vi "communicateUDP.vi"(0 "Communication in":refnum<class "Communication.lvclass">, 1 "Replace Now":bool, 2 "FIRASim?":bool=TRUE, 5 "Robots":T1[](array[typedef]), 7 "isMyTeamYellow":bool, 9 "Address:":string="127.0.0.1", 11 "error in (no error)":errorcluster, 12 "Port:":u16=20011, 13 "grSim replacement":cluster{"robots":T2[], "ball":T3}) -> (4 "Communication out":refnum<class "Communication.lvclass">, 15 "error out":errorcluster)   [LabVIEW 2023, in "Communication.lvclass"]
doc: "Transmits the robots commands to grSim using UDP communication."
uses:
  Communication.lvclass
  Paths/grSim Packet Command UDP Test Folder/grSim/grSim RobotReplacement.ctl
  Paths/grSim Packet Command UDP Test Folder/grSim/grSim_BallReplacement.ctl
  Paths/Convert AI Robot to Robot Command Folder/grSim/grSim Robot Command.ctl
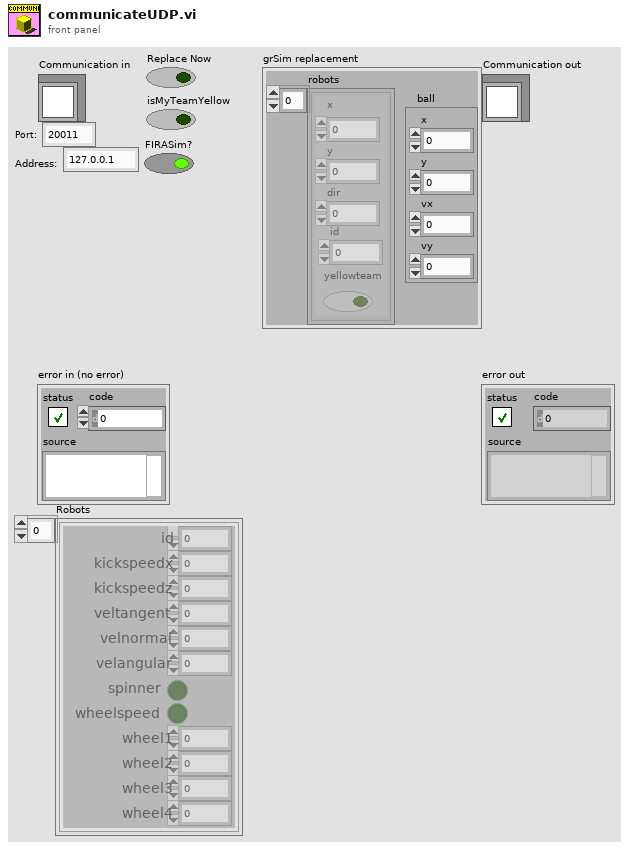
[diagram p1: front panel]
types:
  T1 = typedef "grSim Robot Command.ctl" = cluster{"id":u32, "kickspeedx":sgl, "kickspeedz":sgl, "veltangent":sgl, "velnormal":sgl, "velangular":sgl, "spinner":bool, "wheelspeed":bool, "wheel1":sgl, "wheel2":sgl, "wheel3":sgl, "wheel4":sgl}
  T2 = typedef "grSim RobotReplacement.ctl" = cluster{"x":dbl, "y":dbl, "dir":dbl, "yellowteam":bool, "id":u32}
  T3 = typedef "grSim_BallReplacement.ctl" = cluster{"x":dbl, "y":dbl, "vx":dbl, "vy":dbl}
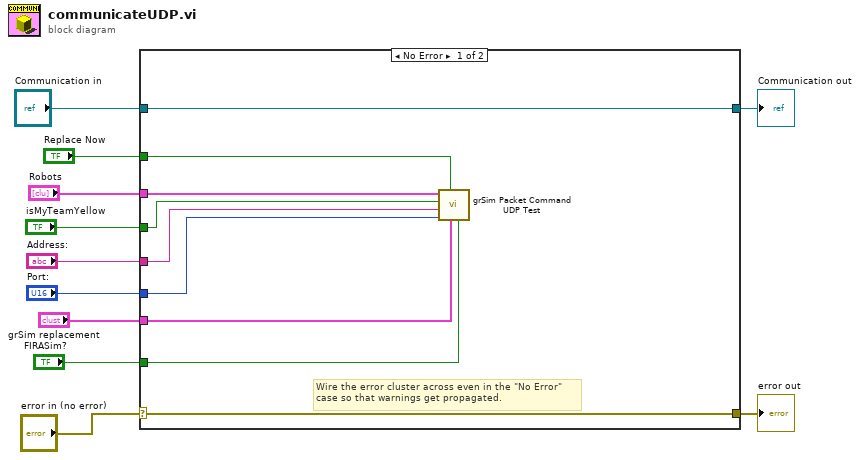
[diagram p0: block diagram]
diagram:
  n1 = case shown="No Error" "error in (no error)" {
    selector: "error in (no error)" -> [w19 w22]
    tunnel: [w19 w22] -> w10
    tunnel: [w20 w21] -> w8
    tunnel: "Communication in" -> [w20 w21]
    tunnel: "Replace Now" -> [w18 _]
    tunnel: "Robots" -> [w17 _]
    tunnel: "isMyTeamYellow" -> [w16 _]
    tunnel: "Address:" -> [w15 _]
    tunnel: "grSim replacement" -> [w14 _]
    tunnel: "Port:" -> [w13 _]
    tunnel: "FIRASim?" -> [w12 _]
    frame No Error {
      # "Wire the error cluster across even in the \"No Error\"\ncase so that warnings get propagated."
      n2 = call "grSim Packet Command UDP Test.vi"("FIRASim?"=w12, "grSim replacement"=w14, "replace ball"=w18, "Port:"=w13, "SSL Vision Address:"=w15, "isteamyellow"=w16, "Robots"=w17) -> ()  [unwired: 5 in]
    }
    frame Error {
    }
  }
  "error out" <- w10
  "Communication out" <- w8
